vi "PH_Cam_BaseClass.PC set Cam on.vi"(0 "i ref in":refnum<vi>, 2 "Cam on":bool, 5 "error in (no error)":errorcluster) -> (14 "i ref out":refnum<vi>, 19 "error out":errorcluster)   [LabVIEW 2014, in "PH_Cam_BaseClass.lvlib"]
doc: "This VI sets a few Attributes and GUI elements."
uses:
  PH_Cam_BaseClass.lvlib
  PH_Common/PH_Common.lvlib
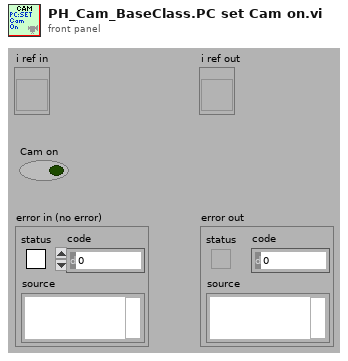
[diagram p1: front panel]
types:
  T1 = typedef "PH_Cam_BaseClass.lvlib/PH_Cam_BaseClass.i attribute.ctl" = cluster{"Gui Refs":T2, "Cam":cluster{"Source Notifier":refnum<notifier>, "Error":errorcluster, "Camera ID":string}, "Images":cluster{"Cam":T3, "Operation":T3, "PSDB":T3}, "Window Image":cluster{"Indicate Image":bool, "Window No.":i32, "Scale Facor":dbl, "Center Cross":bool, "Subtract Backgr":bool, "CoG":bool, "Color Palette":cluster{"Red":u8, "Green":u8, "Blue":u8}[], "Image On":bool}, "Default Prdc Int":i32, "Performance":cluster{"on":bool, "Timestamp Last Frame":i32}, "Histogram":cluster{"on":bool, "Mapping":bool}, "Save Image":cluster{"Save":bool, "File refnum":refnum<file>}, "Setting Service ID":i32, "Screen":cluster{"x-resolution":i16, "y-resolution":i16}, "On":bool, "Constructor finished":bool, "configured":bool}
  T2 = typedef "PH_Cam_BaseClass.lvlib/PH_Cam_BaseClass.GUI Refs.ctl" = cluster{"Frame Rate":refnum<vi>, "Get Frame Rate":refnum<vi>, "Show Image":refnum<vi>, "Get Histogram":refnum<vi>, "Mapping":refnum<vi>, "Histogram":refnum<vi>, "Center Cross":refnum<vi>, "Center of Gravity":refnum<vi>, "Scale Factor [%]":refnum<vi>, "Save Image":refnum<vi>, "Palette":refnum<vi>, "Subtract Background":refnum<vi>, "Cam Error":refnum<vi>, "On":refnum<vi>, "Cam List":refnum<vi>}
  T3 = typedef "IMAQ Image.ctl" = refnum<image>
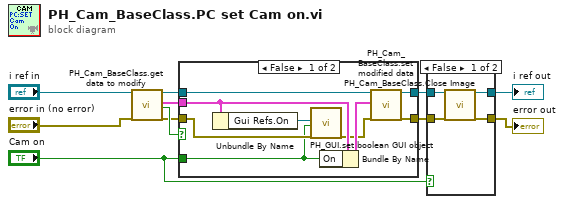
[diagram p0: block diagram]
diagram:
  n1 = call "PH_Cam_BaseClass.get data to modify.vi"("i ref in"="i ref in", "error in (no error)"="error in (no error)") -> ("i ref out"=w9:refnum<vi>, "i attribute"=w10:T1, "timed out"=w11:bool, "error out"=w8:errorcluster)  [unwired: 14 in]
  n2 = case shown="False" w11 {
    tunnel: w8 -> [w15 w21]
    tunnel: [w20 w21] -> w3
    tunnel: w9 -> [w19 w22]
    tunnel: [w18 w22] -> w5
    tunnel: w10 -> [w16 _]
    tunnel: "Cam on" -> [w13 _]
    frame False {
      n3 = Unbundle By Name(w16) -> ("Gui Refs.On"=w12:refnum<vi>)
      n4 = call "PH_GUI.set boolean GUI object.vi"("Boolean Knob GUI Ref"=w12, "Value"=w13, "error in (no error)"=w15) -> ("error out"=w14:errorcluster)  [unwired: 16 in]
      n5 = Bundle By Name(cluster=w16, "On"=w13) -> (w17:T1)
      n6 = call "PH_Cam_BaseClass.set modified data.vi"("i ref in"=w19, "i attribute"=w17, "error in (no error)"=w14) -> ("i ref out"=w18:refnum<vi>, "error out"=w20:errorcluster)  [unwired: 15 in]
    }
    frame True {
    }
  }
  n7 = case shown="False" "Cam on" {
    tunnel: w5 -> [w26 w28]
    tunnel: [w24 w28] -> w4
    tunnel: w3 -> [w25 w27]
    tunnel: [w23 w27] -> w2
    frame False {
      n8 = call "PH_Cam_BaseClass.Close Image.vi"("i ref in"=w26, "error in"=w25) -> ("i ref out"=w24:refnum<vi>, "error out"=w23:errorcluster)  [unwired: 16 in]
    }
    frame True {
    }
  }
  "i ref out" <- w4
  "error out" <- w2
